vi "Read Configuration from File.vi"(8 "error in":errorcluster) -> (0 "error out":errorcluster, 3 "Configuration":T1)   [LabVIEW 2013, in "LVTM.lvlib"]
uses:
  LVTM.lvlib
  Controls_LVTM/LVTM_Config_Info.ctl
  Controls_LVTM/View.ctl
  Controls_LVTM/SharedDataDVR.ctl
  <vilib>/Utility/config.llb/Read Key (String).vi
  <vilib>/Utility/config.llb/Read Key (Boolean).vi
  <vilib>/Utility/config.llb/Read Key (I32).vi
  <vilib>/Utility/config.llb/Read Key (Path).vi
  <vilib>/Utility/config.llb/NI_LVConfig.lvlib
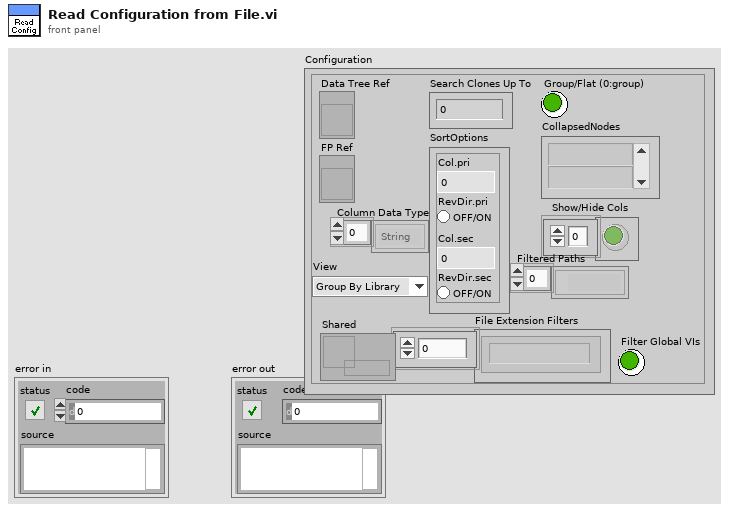
[diagram p1: front panel]
types:
  T1 = typedef "LVTM.lvlib/LVTM_Config_Info.ctl" = cluster{"Data Tree Ref":refnum<vi>, "FP Ref":refnum<vi>, "Column Data Type":enum16{"String", "Numeric"}[], "Search Clones Up To":i32, "SortOptions":cluster{"Col.pri":i32, "RevDir.pri":bool, "Col.sec":i32, "RevDir.sec":bool}, "Group/Flat (0:group)":bool, "CollapsedNodes":string[], "Show/Hide Cols":bool[], "Filtered Paths":path[], "View":T2, "File Extension Filters":string[], "Filter Global VIs":bool, "Shared":refnum<data-value>}
  T2 = typedef "LVTM.lvlib/View.ctl" = enum16{"Group By Library", "Group By Folder", "Flat List"}
  T3 = typedef "NI_LVConfig.lvlib/Config Data RefNum.ctl" = refnum<k1>
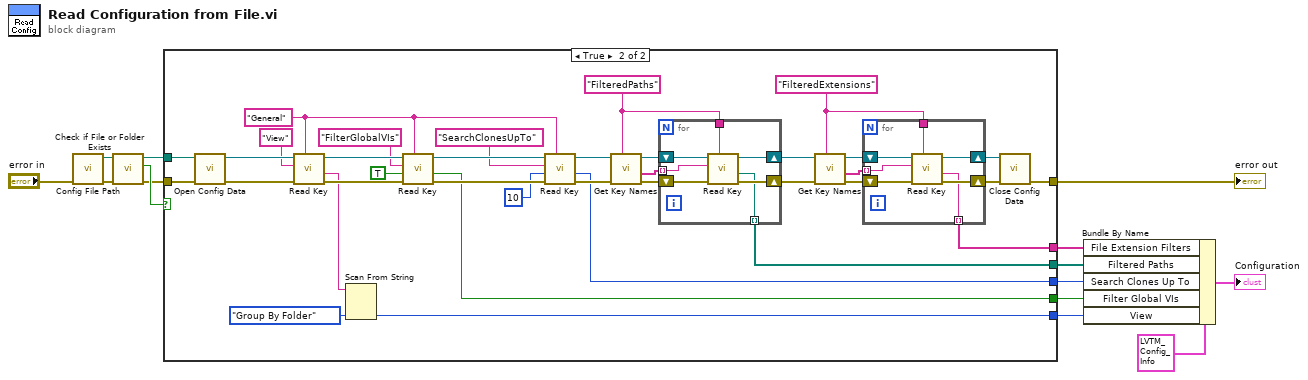
[diagram p0: block diagram]
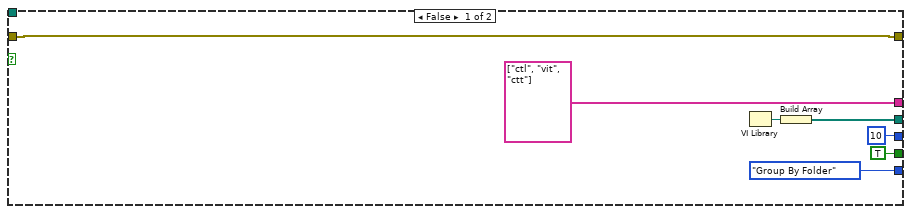
[diagram p2: hidden frame]
diagram:
  n1 = call "Config File Path.vi"("error in"="error in") -> ("error out"=w2:errorcluster, "Config File Path"=w12:path)  [unwired: 9 in]
  n2 = call <vilib>:"Check if File or Folder Exists.vi"("error in (no error)"=w2, "path"=w12) -> ("error out"=w1:errorcluster, "file or folder exists?"=w3:bool, "dup path"=w4:path)  [unwired: 7 in]
  n3 = case shown="True" w3 {
    tunnel: [w15 w57] -> w14
    tunnel: w1 -> [w15 w45]
    tunnel: w4 -> [_ w44]
    tunnel: [View."Group By Folder" ("View") w39] -> w11
    tunnel: [TRUE ("value") w38] -> w10
    tunnel: [10 ("value") w35] -> w9
    tunnel: [w19 w31] -> w8
    tunnel: [string[] ["ctl", "vit", "ctt"] w22] -> w7
    frame False {
      n4 = VI Library() -> (path=w20:path)
      n5 = Build Array(w20) -> (w19:path[])
    }
    frame True {
      w27 = "FilteredExtensions" ("section")
      w42 = "FilteredPaths" ("section")
      w55 = "General" ("section")
      n6 = call <vilib>:"Open Config Data.vi"("error in (no error)"=w45, "configuration file path"=w44) -> ("error out"=w46:errorcluster, "refnum"=w48:T3)  [unwired: 7 in, 1 out]
      n7 = call-poly <vilib>:"Read Key.vi"("section"=w55, "error in (no error)"=w46, "key"="View", "refnum"=w48) -> ("error out"=w51:errorcluster, "value"=w41:string, "refnum out"=w50:T3)  [unwired: 4 in, 1 out]
      n8 = Scan From String(input string=w41, default 1=View."Group By Folder" ("View")) -> (output 1=w39:T2)  [unwired: 3 in, 3 out]
      n9 = call-poly <vilib>:"Read Key.vi"("section"=w55, "error in (no error)"=w51, "default value"=TRUE, "key"="FilterGlobalVIs", "refnum"=w50) -> ("error out"=w54:errorcluster, "value"=w38:bool, "refnum out"=w53:T3)  [unwired: 3 in, 1 out]
      n10 = call-poly <vilib>:"Read Key.vi"("section"=w55, "error in (no error)"=w54, "default value"=10, "key"="SearchClonesUpTo", "refnum"=w53) -> ("error out"=w43:errorcluster, "value"=w35:i32, "refnum out"=w56:T3)  [unwired: 3 in, 1 out]
      n11 = call <vilib>:"Get Key Names.vi"("section"=w42, "error in (no error)"=w43, "refnum"=w56) -> ("error out"=w34:errorcluster, "key names"=w32:string[], "refnum out"=w33:T3)  [unwired: 5 in, 1 out]
      n12 = for {
        shift-right: [w69] -> w26
        shift-left: w33 -> [w70]
        shift-right: [w68] -> w25
        shift-left: w34 -> [w71]
        tunnel: w42 -> [w67]
        tunnel: w32 -> [w66] mode=indexing
        tunnel: [w65] -> w31 mode=indexing
        n13 = call-poly <vilib>:"Read Key.vi"("section"=w67, "error in (no error)"=w71, "key"=w66, "refnum"=w70) -> ("error out"=w68:errorcluster, "value"=w65:path, "refnum out"=w69:T3)  [unwired: 4 in, 1 out]
      }
      n14 = call <vilib>:"Get Key Names.vi"("section"=w27, "error in (no error)"=w25, "refnum"=w26) -> ("error out"=w28:errorcluster, "key names"=w30:string[], "refnum out"=w29:T3)  [unwired: 5 in, 1 out]
      n15 = for {
        shift-right: [w62] -> w24
        shift-left: w29 -> [w63]
        shift-right: [w61] -> w23
        shift-left: w28 -> [w64]
        tunnel: w27 -> [w60]
        tunnel: w30 -> [w59] mode=indexing
        tunnel: [w58] -> w22 mode=indexing
        n16 = call-poly <vilib>:"Read Key.vi"("section"=w60, "error in (no error)"=w64, "key"=w59, "refnum"=w63) -> ("error out"=w61:errorcluster, "value"=w58:string, "refnum out"=w62:T3)  [unwired: 4 in, 1 out]
      }
      n17 = call <vilib>:"Close Config Data.vi"("error in (no error)"=w23, "refnum"=w24) -> ("error out"=w57:errorcluster)  [unwired: 8 in, 1 out]
    }
  }
  "error out" <- w14
  n18 = Bundle By Name(cluster=T1 {"Data Tree Ref"=refnum, "FP Ref"=refnum, "Column Data Type"=[], "Search Clones Up To"=0, "SortOptions"={"Col.pri"=0, "RevDir.pri"=FALSE, "Col.sec"=0, "RevDir.sec"=FALSE}, "Group/Flat (0:group)"=FALSE, "CollapsedNodes"=[], "Show/Hide Cols"=[], "Filtered Paths"=[], "View"=enum."Group By Library", "File Extension Filters"=[], "Filter Global VIs"=FALSE, "Shared"=refnum}, "File Extension Filters"=w7, "Filtered Paths"=w8, "Search Clones Up To"=w9, "Filter Global VIs"=w10, "View"=w11) -> (→"Configuration":T1)
